vi "Sensor Input to line.vi"(6 "Degrees":dbl, 7 "distance front":dbl, 8 "error in (no error)":errorcluster, 9 "sensor y":i32, 10 "Sensor x":i32, 11 "map reference in":refnum<data-value>) -> (0 "error out":errorcluster, 3 "map reference out 2":refnum<data-value>)   [LabVIEW 2012]
uses:
  <vilib>/robotics/Navigation/shared/WorldMap/OccupancyGridWorldMap/NI_Robotics_OccupancyGridWorldMap.lvclass
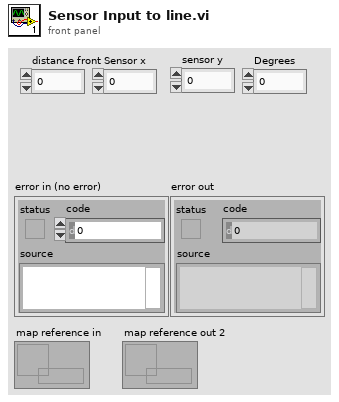
[diagram p1: front panel]
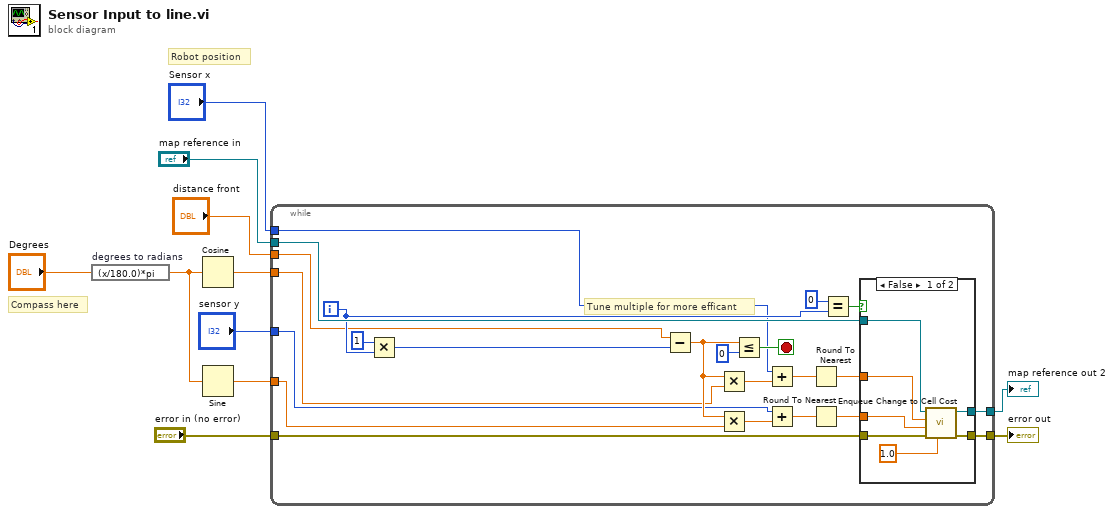
[diagram p0: block diagram]
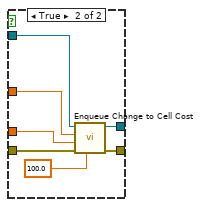
[diagram p2: hidden frame]
diagram:
  # "Robot position"
  # "Compass here"
  n1 = expression code="(x/180.0)*pi" "degrees to radians"("Degrees") -> (w2:dbl)
  n2 = Cosine(x=w2) -> (cos(x)=w3:dbl)
  n3 = Sine(x=w2) -> (sin(x)=w4:dbl)
  n4 = while {
    tunnel: "map reference in" -> [w34]
    tunnel: "error in (no error)" -> [w33]
    tunnel: [w32] -> w10
    tunnel: [w31] -> w11
    tunnel: "sensor y" -> [w13]
    tunnel: "Sensor x" -> [w12]
    tunnel: "distance front" -> [w21]
    tunnel: w4 -> [w18]
    tunnel: w3 -> [w19]
    i -> [w26]
    stop <- w22 stop-if-true
    # "Tune multiple for more efficant"
    n5 = Multiply(x=1, y=w26) -> (x*y=w24:i32)
    n6 = Subtract(x=w21, y=w24) -> (x-y=w20:dbl)
    n7 = Multiply(x=w20, y=w19) -> (x*y=w17:dbl)
    n8 = Multiply(x=w20, y=w18) -> (x*y=w16:dbl)
    n9 = Less Or Equal?(x=w20, y=0) -> (x <= y?=w22:bool)
    n10 = Add(x=w12, y=w17) -> (x+y=w15:dbl)
    n11 = Add(x=w13, y=w16) -> (x+y=w14:dbl)
    n12 = Round To Nearest(number=w15) -> (nearest integer value=w27:dbl)
    n13 = Round To Nearest(number=w14) -> (nearest integer value=w28:dbl)
    n14 = Equal?(x=0, y=w26) -> (x = y?=w29:bool)
    n15 = case shown="False" w29 {
      tunnel: w34 -> [w37 w48]
      tunnel: w33 -> [w38 w47]
      tunnel: [w40 w45] -> w32
      tunnel: [w39 w44] -> w31
      tunnel: w27 -> [w36 w42]
      tunnel: w28 -> [w35 w43]
      frame False {
        n16 = call <vilib>:"Enqueue Change to Cell Cost.vi"("cost"=1.0, "error in (no error)"=w38, "y"=w35, "x"=w36, "map reference in"=w37) -> ("error out"=w39:errorcluster, "map reference out"=w40:refnum<data-value>)  [unwired: 5 in]
      }
      frame True {
        n17 = call <vilib>:"Enqueue Change to Cell Cost.vi"("cost"=100.0, "error in (no error)"=w47, "y"=w43, "x"=w42, "map reference in"=w48) -> ("error out"=w44:errorcluster, "map reference out"=w45:refnum<data-value>)  [unwired: 5 in]
      }
    }
  }
  "map reference out 2" <- w10
  "error out" <- w11
